vi "HEWH Setpoint Temperature Test Requriments.vi"(8 "error in":errorcluster, 11 "UEF Calculated Values Input":T1 {"Data Indexes"."15 sec after Draw Index" format="%#.2f"; "Data Indexes"."15 sec after Draw Timestamp" format="%#.2f"; "Data Indexes"."Test Start Timestamp" format="%.2f"; "Data Indexes"."Test End Timestamp" format="%.2f"; "Data Indexes"."T0 Timestamp" format="%.2f"; "Data Indexes"."Tsf Timestamp" format="%.2f"; "Data Indexes"."Tsu0 Timestamp" format="%.2f"; "Data Indexes"."Tmax1 Timestamp" format="%.2f"; "Data Indexes"."Draw Index Timestamp" format="%#.2f"; "Data Indexes"."Non-Draw Timestamp" format="%#.2f"; "Data Indexes"."Heating Timestamp" format="%#.2f"; "Data Indexes"."Start Energy (BTU-Gas)" format="%.6f"; "Data Indexes"."Start Watt Hours" format="%.6f"; "Static Data"."V - Volume of Wh (True)" format="%.5f"; "Static Data"."T-Ambinet Nominal (°F)" format="%.5f"; "Static Data"."T-Inlet Setpoint (°F)" format="%.5f"; "Static Data"."T-Wh Setpoint (°F)" format="%.5f"; "Sampled Data"."Qe (Wh)" format="%.5f"; "Sampled Data"."Tau stby2 (hr)" format="%.5f"; "Sampled Data"."Tastby2 (°F)" format="%.5f"; "Sampled Data"."Qf (BTU)" format="%.5f"; "Sampled Data"."Qe (BTU)" format="%.5f"; "Sampled Data"."Tmax1 (°F)" format="%.5f"; "Sampled Data"."T0 (°F)" format="%.5f"; "Sampled Data"."Qr (BTU)" format="%.5f"; "Sampled Data"."T 24(°F)" format="%.5f"; "Sampled Data"."T astby(°F)" format="%.5f"; "Sampled Data"."T tstby(°F)" format="%.5f"; "Sampled Data"."T su0(°F)" format="%.5f"; "Sampled Data"."T suf(°F)" format="%.5f"; "Sampled Data"."Tau stby_1 (hr)" format="%.5f"; "Sampled Data"."Qsuf (BTU)" format="%.5f"; "Sampled Data"."Qsu0 (BTU)" format="%.5f"; "Calculated Values"."Draw Bonus Volume (gal)" format="%.6f"; "Calculated Values"."Adjustment Factor" format="%.6f"; "Calculated Values"."T*avg_del(n-1)" format="%.6f"; "Calculated Values"."T*min(n-1)" format="%.6f"; "Calculated Values"."T*avg_del(n)" format="%.6f"; "Calculated Values"."Vn" format="%.6f"; "Calculated Values"."Qdm (BTU)" format="%.6f"; "Calculated Values"."QHWD (BTU)" format="%.6f"; "Calculated Values"."QHW (BTU)" format="%.6f"; "Calculated Values"."UEF" format="%.6f"; "Calculated Values"."QHW67 (BTU)" format="%.6f"; "Calculated Values"."Qda (BTU)" format="%.6f"; "Calculated Values"."Qd (BTU)" format="%.6f"; "Calculated Values"."Q (BTU)" format="%.6f"; "Calculated Values"."UA (BTU/(hr*F))" format="%.6f"; "Calculated Values"."Qhr (BTU/hr)" format="%.6f"; "Calculated Values"."Qstby (BTU)" format="%.6f"; "Calculated Values"."nu_r" format="%.6f"; "Calculated Values"."CpUEF (BTU/(lb*F))" format="%.6f"; "Calculated Values"."rho_nu (lb/gal)" format="%.6f"; "Calculated Values"."V1- Vol (Gal)" format="%.6f"; "Calculated Values"."M cluster mass removed (lb)" format="%.6f"; "Calculated Values"."Cp theoretical (BTU/(lbm °F))" format="%.6f"; "Calculated Values"."Tin1 - Mean Inlet 1st Cluster (°F)" format="%.6f"; "Calculated Values"."Tdel1-Mean Outlet 1st Cluster(°F)" format="%.6f"; "Calculated Values"."Cp 24 (BTU/(lb*F))" format="%.6f"; "Calculated Values"."Cp standby (BTU/(lb*F))" format="%.6f"; "Calculated Values"."Cp2 (BTU/(lb*F))" format="%.6f"; "Calculated Values"."Cp1 (BTU/(lb*F))" format="%.6f"; "Calculated Values"."rho 24 (lb/gal)" format="%.6f"; "Calculated Values"."rho standby (lb/gal)" format="%.6f"; "Calculated Values"."rho 2 (lb/gal)" format="%.6f"; "Calculated Values"."Density of cold water All (lbm/gal)" format="%#.3g"; "Calculated Values"."CpHW (BTU/(lbm °F))" format="%#.3g"; "Calculated Values"."Density of hot water All (lbm/gal)" format="%#.3g"; "Calculated Values"."Mass of water All (lbm)" format="%#.3f"}) -> (0 "error out":errorcluster, 3 "UEF Calculated Values Output":T1 {"Data Indexes"."15 sec after Draw Index" format="%#.2f"; "Data Indexes"."15 sec after Draw Timestamp" format="%#.2f"; "Data Indexes"."Test Start Timestamp" format="%.2f"; "Data Indexes"."Test End Timestamp" format="%.2f"; "Data Indexes"."T0 Timestamp" format="%.2f"; "Data Indexes"."Tsf Timestamp" format="%.2f"; "Data Indexes"."Tsu0 Timestamp" format="%.2f"; "Data Indexes"."Tmax1 Timestamp" format="%.2f"; "Data Indexes"."Draw Index Timestamp" format="%#.2f"; "Data Indexes"."Non-Draw Timestamp" format="%#.2f"; "Data Indexes"."Heating Timestamp" format="%#.2f"; "Data Indexes"."Start Energy (BTU-Gas)" format="%.6f"; "Data Indexes"."Start Watt Hours" format="%.6f"; "Static Data"."V - Volume of Wh (True)" format="%.5f"; "Static Data"."T-Ambinet Nominal (°F)" format="%.5f"; "Static Data"."T-Inlet Setpoint (°F)" format="%.5f"; "Static Data"."T-Wh Setpoint (°F)" format="%.5f"; "Sampled Data"."Qe (Wh)" format="%.5f"; "Sampled Data"."Tau stby2 (hr)" format="%.5f"; "Sampled Data"."Tastby2 (°F)" format="%.5f"; "Sampled Data"."Qf (BTU)" format="%.5f"; "Sampled Data"."Qe (BTU)" format="%.5f"; "Sampled Data"."Tmax1 (°F)" format="%.5f"; "Sampled Data"."T0 (°F)" format="%.5f"; "Sampled Data"."Qr (BTU)" format="%.5f"; "Sampled Data"."T 24(°F)" format="%.5f"; "Sampled Data"."T astby(°F)" format="%.5f"; "Sampled Data"."T tstby(°F)" format="%.5f"; "Sampled Data"."T su0(°F)" format="%.5f"; "Sampled Data"."T suf(°F)" format="%.5f"; "Sampled Data"."Tau stby_1 (hr)" format="%.5f"; "Sampled Data"."Qsuf (BTU)" format="%.5f"; "Sampled Data"."Qsu0 (BTU)" format="%.5f"; "Calculated Values"."Draw Bonus Volume (gal)" format="%.6f"; "Calculated Values"."Adjustment Factor" format="%.6f"; "Calculated Values"."T*avg_del(n-1)" format="%.6f"; "Calculated Values"."T*min(n-1)" format="%.6f"; "Calculated Values"."T*avg_del(n)" format="%.6f"; "Calculated Values"."Vn" format="%.6f"; "Calculated Values"."Qdm (BTU)" format="%.6f"; "Calculated Values"."QHWD (BTU)" format="%.6f"; "Calculated Values"."QHW (BTU)" format="%.6f"; "Calculated Values"."UEF" format="%.6f"; "Calculated Values"."QHW67 (BTU)" format="%.6f"; "Calculated Values"."Qda (BTU)" format="%.6f"; "Calculated Values"."Qd (BTU)" format="%.6f"; "Calculated Values"."Q (BTU)" format="%.6f"; "Calculated Values"."UA (BTU/(hr*F))" format="%.6f"; "Calculated Values"."Qhr (BTU/hr)" format="%.6f"; "Calculated Values"."Qstby (BTU)" format="%.6f"; "Calculated Values"."nu_r" format="%.6f"; "Calculated Values"."CpUEF (BTU/(lb*F))" format="%.6f"; "Calculated Values"."rho_nu (lb/gal)" format="%.6f"; "Calculated Values"."V1- Vol (Gal)" format="%.6f"; "Calculated Values"."M cluster mass removed (lb)" format="%.6f"; "Calculated Values"."Cp theoretical (BTU/(lbm °F))" format="%.6f"; "Calculated Values"."Tin1 - Mean Inlet 1st Cluster (°F)" format="%.6f"; "Calculated Values"."Tdel1-Mean Outlet 1st Cluster(°F)" format="%.6f"; "Calculated Values"."Cp 24 (BTU/(lb*F))" format="%.6f"; "Calculated Values"."Cp standby (BTU/(lb*F))" format="%.6f"; "Calculated Values"."Cp2 (BTU/(lb*F))" format="%.6f"; "Calculated Values"."Cp1 (BTU/(lb*F))" format="%.6f"; "Calculated Values"."rho 24 (lb/gal)" format="%.6f"; "Calculated Values"."rho standby (lb/gal)" format="%.6f"; "Calculated Values"."rho 2 (lb/gal)" format="%.6f"; "Calculated Values"."Density of cold water All (lbm/gal)" format="%#.3g"; "Calculated Values"."CpHW (BTU/(lbm °F))" format="%#.3g"; "Calculated Values"."Density of hot water All (lbm/gal)" format="%#.3g"; "Calculated Values"."Mass of water All (lbm)" format="%#.3f"})   [LabVIEW 2023]
uses:
  Type Definitions/UEF Constants.ctl
  Type Definitions/HEWH Draw Stats.ctl
  Type Definitions/HEWH FHR Draw Type.ctl
  Type Definitions/FHR Bins.ctl
  Type Definitions/HEWH Meter Type.ctl
  <vilib>/Utility/error.llb/whitespace.ctl
  <vilib>/Utility/error.llb/Trim Whitespace One-Sided.vi
panel:
  out "Array":string[][](array[string])
  out "ToutletMin":dbl[](array[numeric])
  out "ToutletMax":dbl[](array[numeric])
  # "FHR"
  # "FHR"
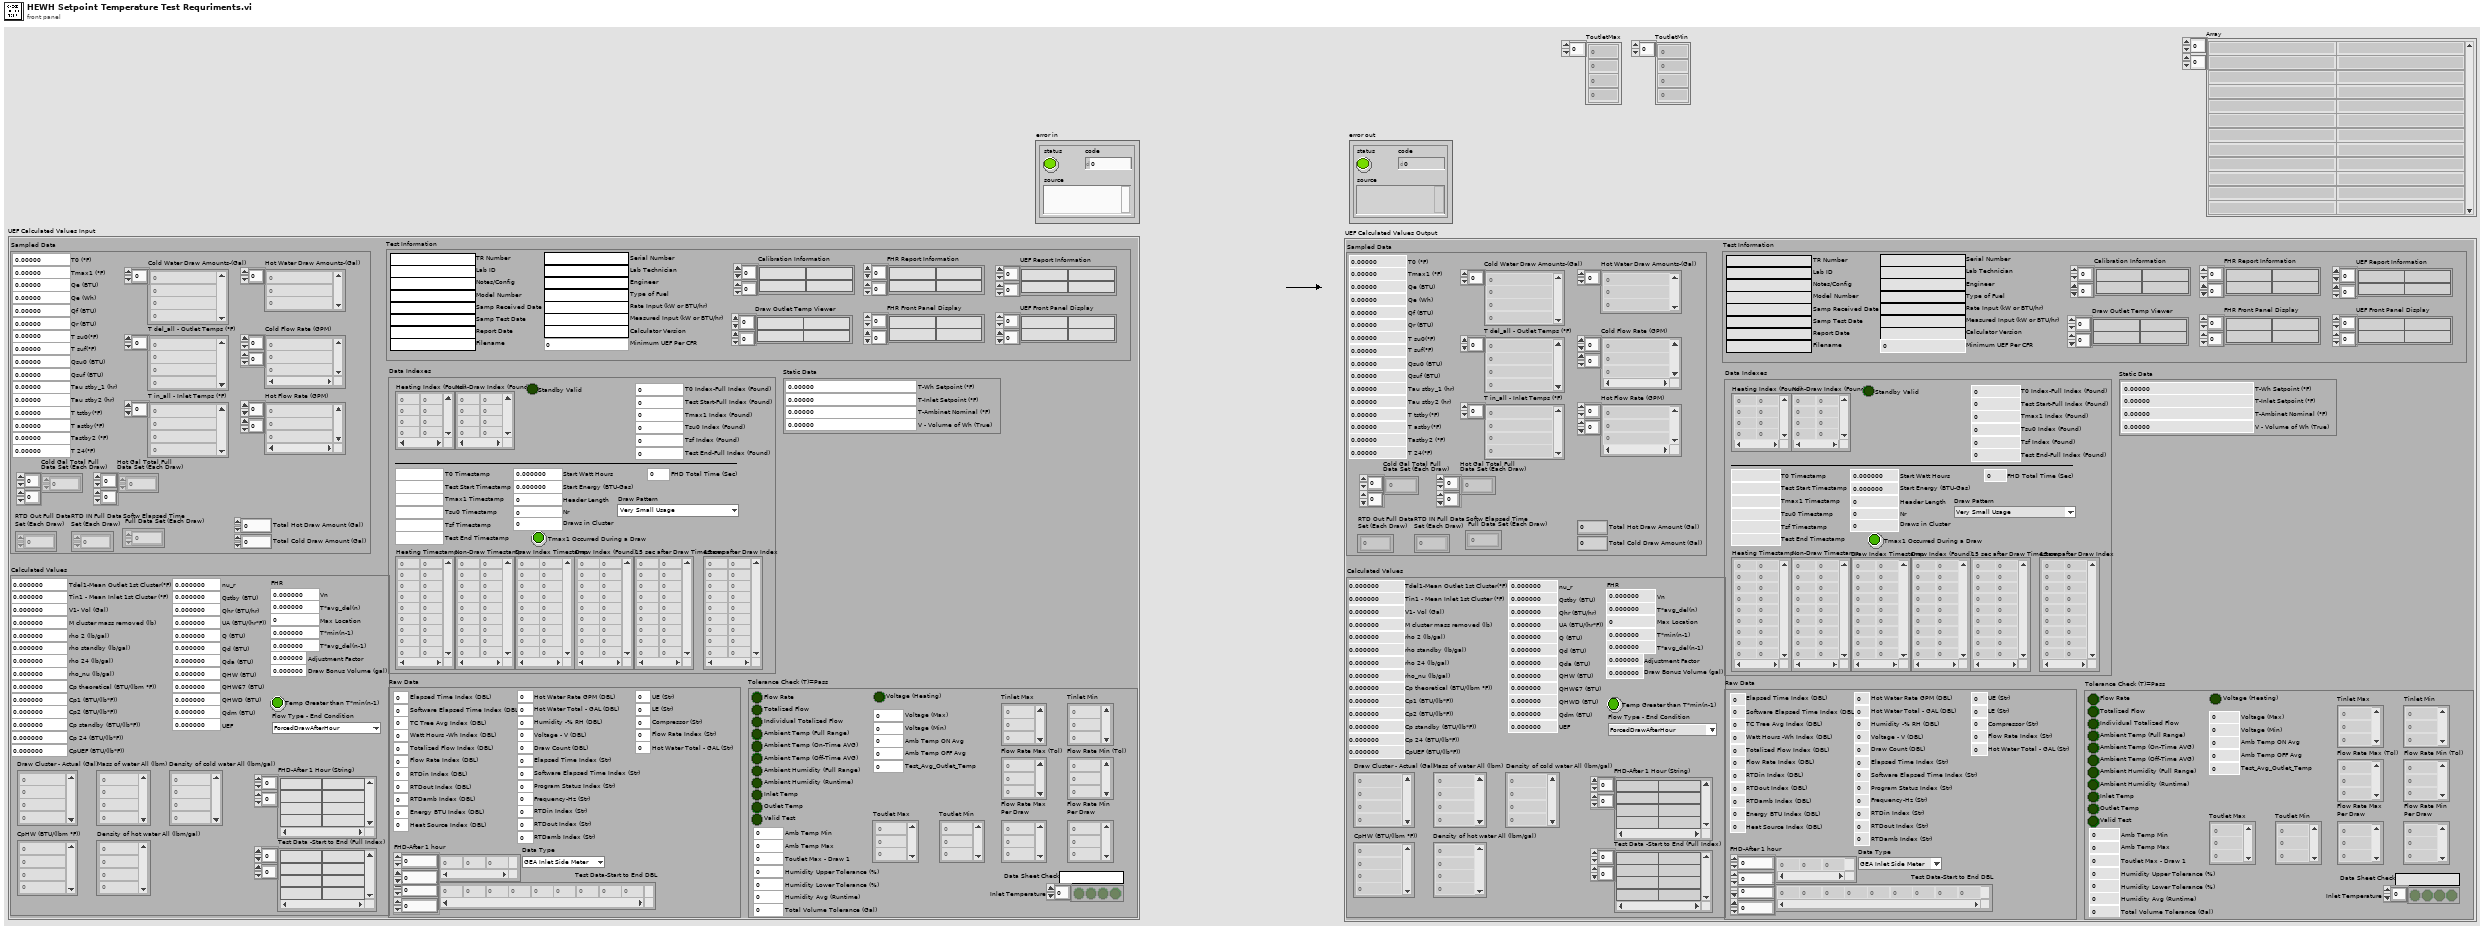
[diagram p1: front panel]
types:
  T1 = typedef "UEF Constants.ctl" = cluster{"Calculated Values":T2, "Sampled Data":cluster{"Cold Water Draw Amounts-(Gal)":dbl[], "T del_all - Outlet Temps (°F)":dbl[], "T in_all - Inlet Temps (°F)":dbl[], "Qsu0 (BTU)":dbl, "Qsuf (BTU)":dbl, "Tau stby_1 (hr)":dbl, "T suf(°F)":dbl, "T su0(°F)":dbl, "T tstby(°F)":dbl, "T astby(°F)":dbl, "T 24(°F)":dbl, "Qr (BTU)":dbl, "T0 (°F)":dbl, "Tmax1 (°F)":dbl, "Qe (BTU)":dbl, "Qf (BTU)":dbl, "Tastby2 (°F)":dbl, "RTD Out Full Data\nSet (Each Draw)":dbl[][], "RTD IN Full Data\nSet (Each Draw)":dbl[][], "Tau stby2 (hr)":dbl, "Hot Water Draw Amounts-(Gal)":dbl[], "Cold Flow Rate (GPM)":dbl[][], "Hot Flow Rate (GPM)":dbl[][], "Softw Elapsed Time\n Full Data Set (Each Draw)":dbl[][], "Cold Gal Total Full\nData Set (Each Draw)":dbl[][], "Total Hot Draw Amount (Gal) ":dbl, "Total Cold Draw Amount (Gal)":dbl, "Qe (Wh)":dbl, "Hot Gal Total Full\nData Set (Each Draw)":dbl[][]}, "Static Data":cluster{"T-Wh Setpoint (°F)":dbl, "T-Inlet Setpoint (°F)":dbl, "T-Ambinet Nominal (°F)":dbl, "V - Volume of Wh (True)":dbl}, "Data Indexes":cluster{"Test Start-Full Index (Found)":i32, "Header Length":i32, "Draw Index (Found)":i32[][], "Nr":i32, "Start Watt Hours":dbl, "Tsu0 Index (Found)":i32, "Tsf Index (Found)":i32, "Start Energy (BTU-Gas)":dbl, "Draws in Cluster":i32, "T0 Index-Full Index (Found)":i32, "Non-Draw Index (Found)":i32[][], "Tmax1 Index (Found)":i32, "Test End-Full Index (Found)":i32, "Heating Index (Found)":i32[][], "Heating Timestamp":dbl[][], "Non-Draw Timestamp":dbl[][], "Draw Index Timestamp":dbl[][], "Tmax1 Timestamp":dbl, "Tsu0 Timestamp":dbl, "Tsf Timestamp":dbl, "T0 Timestamp":dbl, "Test End Timestamp":dbl, "Test Start Timestamp":dbl, "15 sec after Draw Timestamp":dbl[][], "15 sec after Draw Index":dbl[][], "Tmax1 Occurred During a Draw":bool, "FHD Total Time (Sec)":dbl, "Draw Pattern":T4, "Standby Valid":bool}, "Raw Data":cluster{"Elapsed Time Index (DBL)":i32, "Software Elapsed Time Index (DBL)":i32, "TC Tree Avg Index (DBL)":i32, "Watt Hours -Wh Index (DBL)":i32, "Energy BTU Index (DBL)":i32, "Totalized Flow Index (DBL)":i32, "Flow Rate Index (DBL)":i32, "Program Status Index (Str)":i32, "RTDin Index (DBL)":i32, "RTDout Index (DBL)":i32, "RTDamb Index (DBL)":i32, "Test Data-Start to End DBL":dbl[][], "Data Type":T5, "Heat Source Index (DBL)":i32, "Hot Water Rate GPM (DBL)":i32, "Hot Water Total - GAL (DBL)":i32, "FHD-After 1 hour":dbl[][], "Humidity -% RH (DBL)":i32, "Voltage - V (DBL)":i32, "Draw Count (DBL)":i32, "Elapsed Time Index (Str)":i32, "Software Elapsed Time Index (Str)":i32, "Frequency-Hz (Str)":i32, "RTDin Index (Str)":i32, "RTDout Index (Str)":i32, "RTDamb Index (Str)":i32, "UE (Str)":i32, "LE (Str)":i32, "Compressor (Str)":i32, "Flow Rate Index (Str)":i32, "Hot Water Total - GAL (Str)":i32}, "Tolerance Check (T)=Pass":cluster{"Flow Rate":bool, "Totalized Flow":bool, "Ambient Temp (Full Range)":bool, "Ambient Humidity (Full Range)":bool, "Inlet Temp":bool, "Outlet Temp":bool, "Valid Test":bool, "Individual Totalized Flow":bool, "Data Sheet Check":string, "Inlet Temperature":bool[], "Tinlet Max":dbl[], "Tinlet Min":dbl[], "Flow Rate Max (Tol)":dbl[], "Flow Rate Min (Tol)":dbl[], "Amb Temp Max":dbl, "Amb Temp Min":dbl, "Toutlet Max - Draw 1":dbl, "Humidity Upper Tolerance (%)":dbl, "Total Volume Tolerance (Gal)":dbl, "Humidity Lower Tolerance (%)":dbl, "Flow Rate Max\nPer Draw":dbl[], "Flow Rate Min\nPer Draw":dbl[], "Ambient Humidity (Runtime)":bool, "Humidity Avg (Runtime)":dbl, "Ambient Temp (On-Time AVG)":bool, "Ambient Temp (Off-Time AVG)":bool, "Amb Temp OFF Avg":dbl, "Amb Temp ON Avg":dbl, "Voltage (Heating)":bool, "Voltage (Min)":dbl, "Voltage (Max)":dbl, "Toutlet Max":dbl[], "Toutlet Min":dbl[], "Test_Avg_Outlet_Temp":dbl}, "Test Information":cluster{"TR Number":string, "Lab ID":string, "Notes/Config":string, "Model Number":string, "Serial Number":string, "Lab Technician":string, "Engineer":string, "Type of Fuel":string, "Samp Received Date":string, "Samp Test Date":string, "Report Date":string, "Rate Input (kW or BTU/hr)":string, "Measured Input (kW or BTU/hr)":string, "Filename":string, "Calibration Information":string[][], "Calculator Version":string, "Minimum UEF Per CFR":dbl, "UEF Report Information":string[][], "FHR Report Information":string[][], "FHR Front Panel Display":string[][], "UEF Front Panel Display":string[][], "Draw Outlet Temp Viewer":string[][]}}
  T2 = typedef "HEWH Draw Stats.ctl" = cluster{"Draw Cluster - Actual (Gal)":dbl[], "Mass of water All (lbm)":dbl[], "Density of hot water All (lbm/gal)":dbl[], "CpHW (BTU/(lbm °F))":dbl[], "rho 2 (lb/gal)":dbl, "rho standby (lb/gal)":dbl, "rho 24 (lb/gal)":dbl, "Cp1 (BTU/(lb*F))":dbl, "Cp2 (BTU/(lb*F))":dbl, "Cp standby (BTU/(lb*F))":dbl, "Cp 24 (BTU/(lb*F))":dbl, "nu_r":dbl, "Qstby (BTU)":dbl, "Qhr (BTU/hr)":dbl, "UA (BTU/(hr*F))":dbl, "Q (BTU)":dbl, "Qd (BTU)":dbl, "Qda (BTU)":dbl, "QHW67 (BTU)":dbl, "UEF":dbl, "Tdel1-Mean Outlet 1st Cluster(°F)":dbl, "Tin1 - Mean Inlet 1st Cluster (°F)":dbl, "Cp theoretical (BTU/(lbm °F))":dbl, "M cluster mass removed (lb)":dbl, "V1- Vol (Gal)":dbl, "Test Data -Start to End (Full Index)":string[][], "rho_nu (lb/gal)":dbl, "Density of cold water All (lbm/gal)":dbl[], "CpUEF (BTU/(lb*F))":dbl, "QHW (BTU)":dbl, "QHWD (BTU)":dbl, "Qdm (BTU)":dbl, "FHD-After 1 Hour (String)":string[][], "Vn":dbl, "T*avg_del(n)":dbl, "Max Location":i32, "T*min(n-1)":dbl, "T*avg_del(n-1)":dbl, "Temp Greater than T*min(n-1)":bool, "Adjustment Factor":dbl, "Draw Bonus Volume (gal)":dbl, "Flow Type - End Condition":T3}
  T3 = typedef "HEWH FHR Draw Type.ctl" = enum16{"ForcedDrawAfterHour", "HeatingCutoffBeforeHour"}
  T4 = typedef "FHR Bins.ctl" = enum16{"Very Small Usage", "Low Usage", "Medium Usage", "High Usage", "Undefined"}
  T5 = typedef "HEWH Meter Type.ctl" = enum16{"GEA Inlet Side Meter", "GEA Outlet Side Meter", "CSA Inlet Side Meter"}
  T6 = typedef "whitespace.ctl" = u16
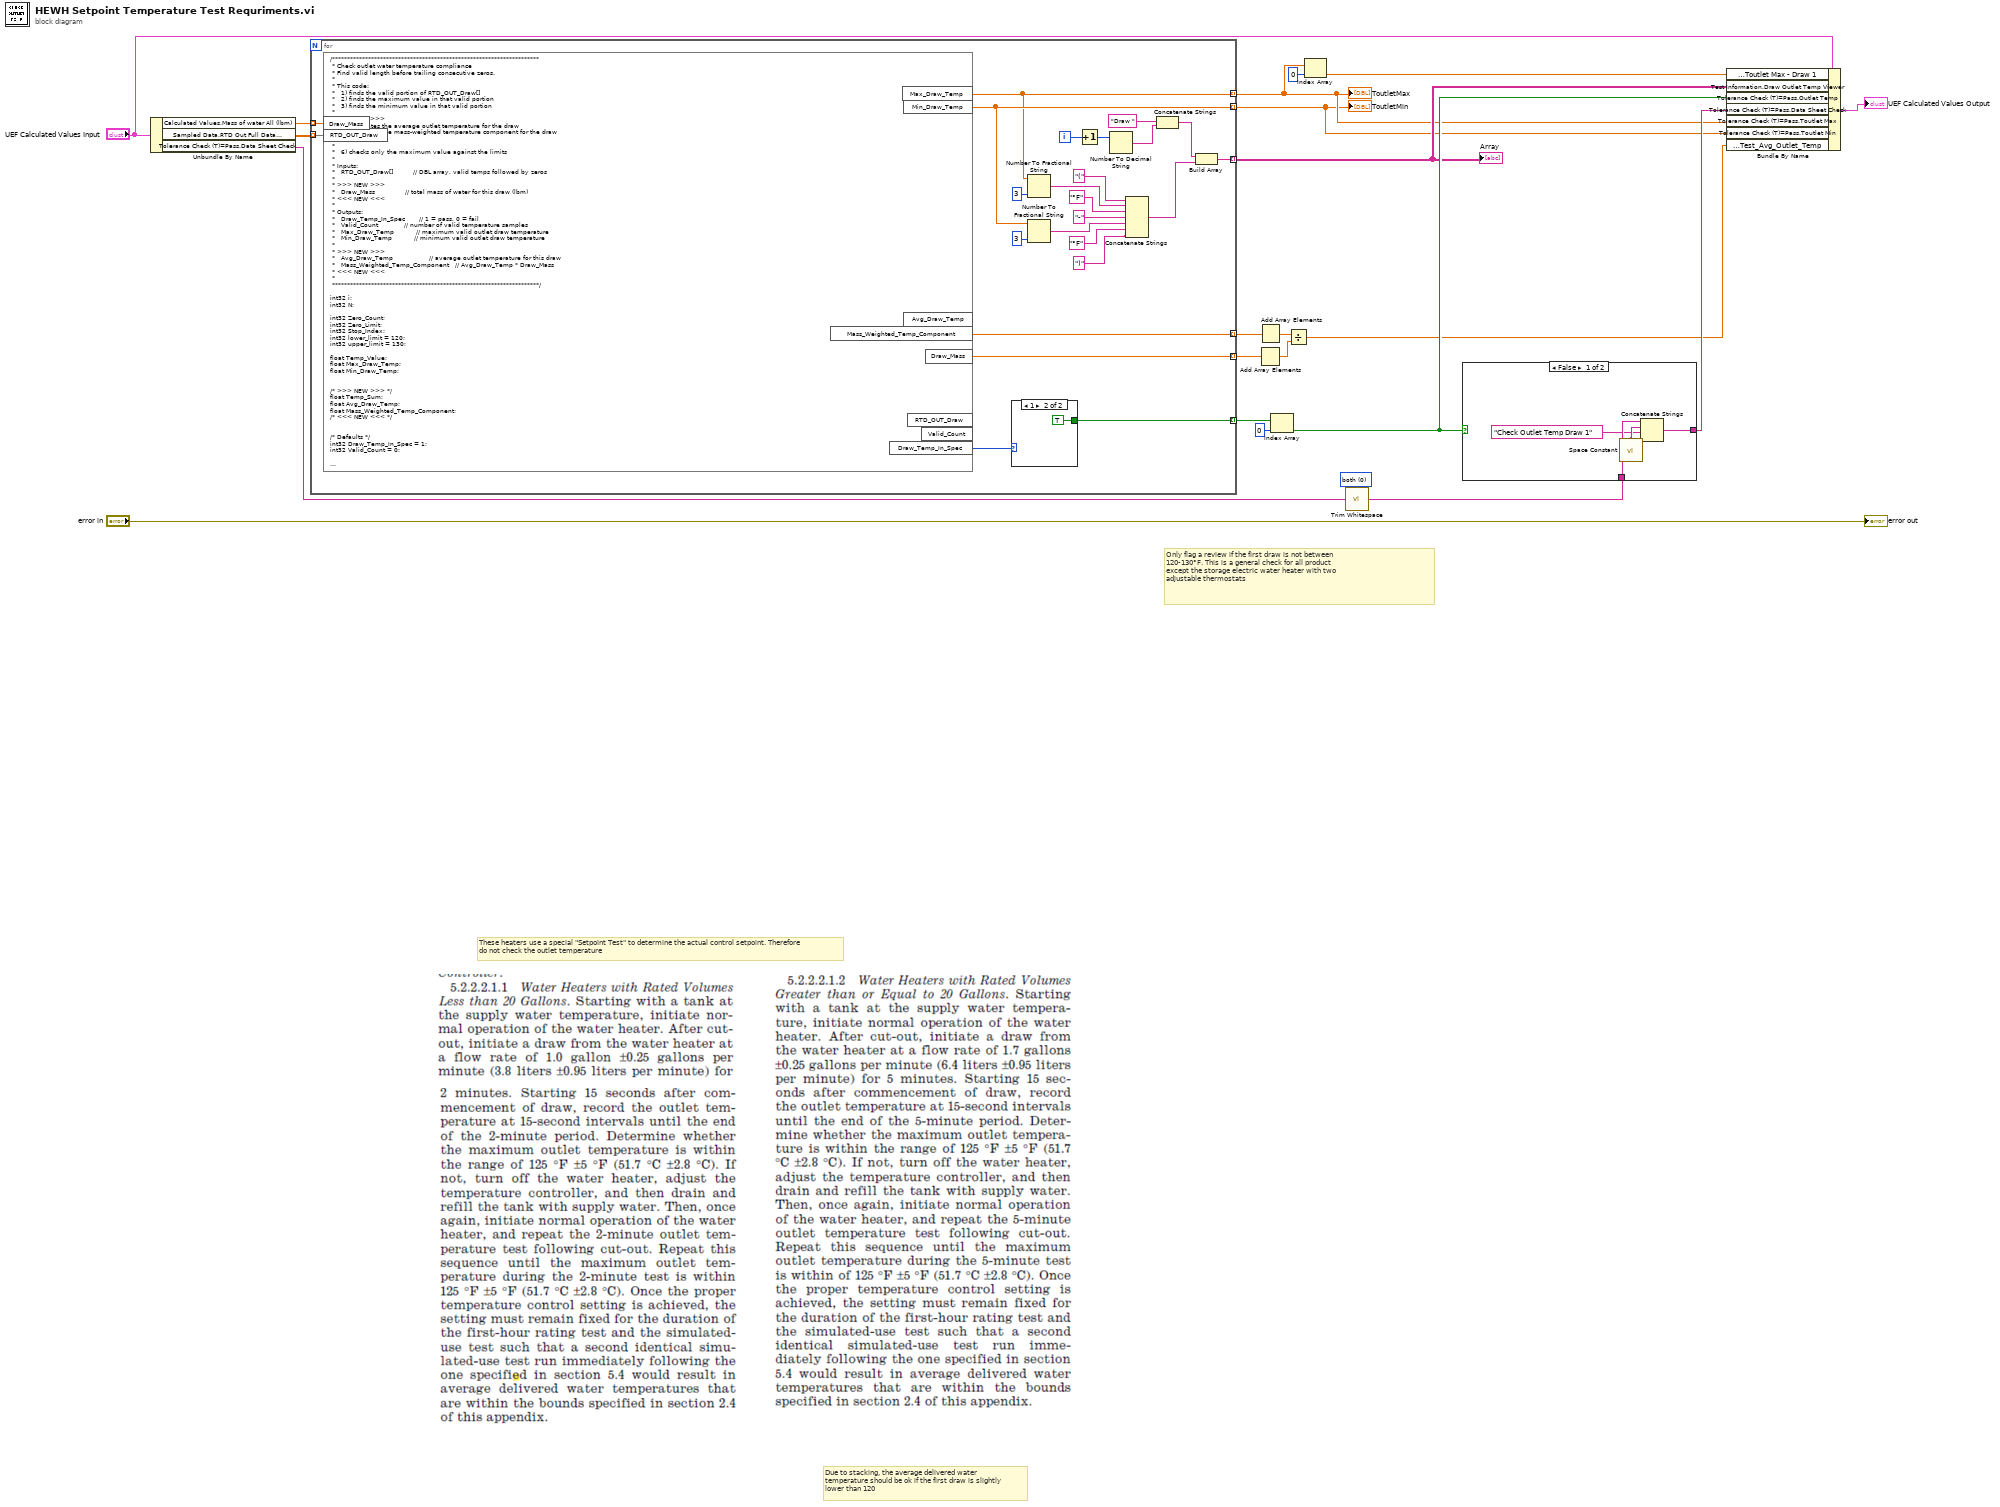
[diagram p0: block diagram]
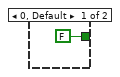
[diagram p3: hidden frame]
diagram:
  w11 = T6 0 items=["both", "start of string", "end of string"] ("location (both)")
  # "Only flag a review if the first draw is not between\n120-130°F. This is a general check for all product\nexcept the storage electric water heater with two \nadjustable thermostats"
  # "These heaters use a special \"Setpoint Test\" to determine the actual control setpoint. Therefore\ndo not check the outlet temperature"
  # "Due to stacking, the average delivered water\ntemperature should be ok if the first draw is slightly \nlower than 120"
  n1 = Unbundle By Name("UEF Calculated Values Input") -> ("Calculated Values.Mass of water All (lbm)"=w6:dbl[], "Sampled Data.RTD Out Full Data\nSet (Each Draw)"=w18:dbl[][], "Tolerance Check (T)=Pass.Data Sheet Check"=w13:string)
  n2 = for {
    tunnel: w18 -> [w30] mode=indexing
    tunnel: [w35] -> w9 mode=indexing
    tunnel: [w28] -> w20 mode=indexing
    tunnel: [w26] -> w8 mode=indexing
    tunnel: [w27] -> w7 mode=indexing
    tunnel: w6 -> [w25] mode=indexing
    tunnel: [w24] -> w5 mode=indexing
    tunnel: [w23] -> w3 mode=indexing
    i -> [w34]
    n3 = formula code="/*********************************************************************\n * Check outlet water temperature compliance\n * Find valid length before trailing consecutive zeros.\n *\n * This code:\n *   1) finds the valid portion of RTD_OUT_Draw[]\n *   2) finds the maximum value in that valid portion\n *   3) finds the minimum value in that valid portion\n *\n * >>> NEW >>>\n *   4) calculates the average outlet temperature for the draw\n *   5) calculates the mass-weighted temperature component for the draw\n * <<< NEW <<<\n *\n *   6) checks only the maximum value against the limits\n *\n * Inputs:\n *   RTD_OUT_Draw[]          // DBL array, valid temps followed by zeros\n *\n * >>> NEW >>>\n *   Draw_Mass               // total mass of water for this draw (lbm)\n * <<< NEW <<<\n *\n * Outputs:\n *   Draw_Temp_In_Spec       // 1 = pass, 0 = fail\n *   Valid_Count             // number of valid temperature samples\n *   Max_Draw_Temp           // maximum valid outlet draw temperature\n *   Min_Draw_Temp           // minimum valid outlet draw temperature\n *\n * >>> NEW >>>\n *   Avg_Draw_Temp                  // average outlet temperature for this draw\n *   Mass_Weighted_Temp_Component   // Avg_Draw_Temp * Draw_Mass\n * <<< NEW <<<\n *\n *********************************************************************/\n\nint32 i;\nint32 N;\n\nint32 Zero_Count;\nint32 Zero_Limit;\nint32 Stop_Index;\nint32 lower_limit = 120;\nint32 upper_limit = 130;\n\nfloat Temp_Value;\nfloat Max_Draw_Temp;\nfloat Min_Draw_Temp;\n\n\n/* >>> NEW >>> */\nfloat Temp_Sum;\nfloat Avg_Draw_Temp;\nfloat Mass_Weighted_Temp_Component;\n/* <<< NEW <<< */\n\n\n/* Defaults */\nint32 Draw_Temp_In_Spec = 1;\nint32 Valid_Count = 0;\n\n\n/* >>> NEW >>> */\nTemp_Sum = 0.0;\nAvg_Draw_Temp = 0.0;\nMass_Weighted_Temp_Component = 0.0;\n/* <<< NEW <<< */\n\n\nZero_Count = 0;\nZero_Limit = 3;        /* Stop after 3 consecutive zeros */\nStop_Index = -1;\n\nN = sizeOfDim(RTD_OUT_Draw, 0);\n\n\n/*\n * Find the start of the trailing zero section.\n */\nfor (i = 0; i < N; i++)\n{\n    Temp_Value = RTD_OUT_Draw[i];\n\n    if (Temp_Value == 0.0)\n    {\n        Zero_Count += 1;\n\n        if (Zero_Count >= Zero_Limit)\n        {\n            /*\n             * i is the index of the third zero.\n             * Last valid temp is before the zero run.\n             */\n            Stop_Index = i - Zero_Limit;\n            break;\n        }\n    }\n    else\n    {\n        Zero_Count = 0;\n    }\n}\n\n\n/*\n * If no trailing zero section was found, use the full array.\n */\nif (Stop_Index < 0)\n{\n    Stop_Index = N - 1;\n}\n\n\n/*\n * Number of valid samples to keep.\n */\nValid_Count = Stop_Index + 1;\n\n\n/*\n * Find the maximum and minimum valid temperatures.\n * Only the maximum temperature is checked against the limits.\n */\nif (Valid_Count > 0)\n{\n    Max_Draw_Temp = RTD_OUT_Draw[0];\n    Min_Draw_Temp = RTD_OUT_Draw[0];\n\n\n    /* >>> NEW >>> */\n    /*\n     * Start the temperature sum with the first valid sample.\n     */\n    Temp_Sum = RTD_OUT_Draw[0];\n    /* <<< NEW <<< */\n\n\n    for (i = 1; i < Valid_Count; i++)\n    {\n        Temp_Value = RTD_OUT_Draw[i];\n\n\n        /* >>> NEW >>> */\n        /*\n         * Add each valid temperature sample to the running sum.\n         */\n        Temp_Sum += Temp_Value;\n        /* <<< NEW <<< */\n\n\n        if (Temp_Value > Max_Draw_Temp)\n        {\n            Max_Draw_Temp = Temp_Value;\n        }\n\n        if (Temp_Value < Min_Draw_Temp)\n        {\n            Min_Draw_Temp = Temp_Value;\n        }\n    }\n\n\n    /* >>> NEW >>> */\n    /*\n     * Calculate average outlet temperature for this draw.\n     */\n    Avg_Draw_Temp = Temp_Sum / Valid_Count;\n\n\n    /*\n     * Calculate this draw's contribution to the whole-test\n     * mass-weighted average outlet temperature.\n     *\n     * Final calculation outside the For Loop:\n     *\n     *                       Sum(Mass_Weighted_Temp_Component)\n     * Test_Avg_Temp = -----------------------------------------\n     *                              Sum(Draw_Mass)\n     */\n    if (Draw_Mass > 0.0)\n    {\n        Mass_Weighted_Temp_Component =\n            Avg_Draw_Temp * Draw_Mass;\n    }\n    else\n    {\n        Mass_Weighted_Temp_Component = 0.0;\n    }\n    /* <<< NEW <<< */\n\n\n    if (Max_Draw_Temp < lower_limit || Max_Draw_Temp > upper_limit)\n    {\n        Draw_Temp_In_Spec = 0;\n    }\n}\nelse\n{\n    Max_Draw_Temp = 0.0;\n    Min_Draw_Temp = 0.0;\n\n\n    /* >>> NEW >>> */\n    Avg_Draw_Temp = 0.0;\n    Mass_Weighted_Temp_Component = 0.0;\n    /* <<< NEW <<< */\n\n\n    Draw_Temp_In_Spec = 0;\n}"("RTD_OUT_Draw"=w30, "Draw_Mass"=w25) -> ("Draw_Temp_In_Spec"=w29:i32, "Max_Draw_Temp"=w26:dbl, "Min_Draw_Temp"=w27:dbl, "Mass_Weighted_Temp_Component"=w24:dbl, "Draw_Mass"=w23:dbl)  [unwired: 3 out]
    n4 = case shown="1" w29 {
      tunnel: [FALSE TRUE] -> w28
      frame 0, Default {
      }
      frame 1 {
      }
    }
    n5 = Number To Fractional String(number=w26, precision (6)=i16 3) -> (F-format string=w46:string)  [unwired: 2 in]
    n6 = Number To Fractional String(number=w27, precision (6)=i16 3) -> (F-format string=w44:string)  [unwired: 2 in]
    n7 = Increment(x=w34) -> (x+1=w33:i32)
    n8 = Number To Decimal String(number=w33) -> (decimal integer string=w38:string)  [unwired: 1 in]
    n9 = Concatenate Strings("(" ("string"), w46, "°F" ("string"), "-" ("string"), w44, "°F" ("string"), ")" ("string")) -> (w36:string)
    n10 = Concatenate Strings("Draw ", w38) -> (w37:string)
    n11 = Build Array(w37, w36) -> (w35:string[])
  }
  "ToutletMax" <- w8
  "ToutletMin" <- w7
  "Array" <- w9
  n12 = Add Array Elements(numeric array=w3) -> (sum=w2:dbl)
  n13 = Add Array Elements(numeric array=w5) -> (sum=w4:dbl)
  n14 = Index Array(array=w20, index=0) -> (element=w10:bool)
  n15 = Divide(x=w4, y=w2) -> (x/y=w1:dbl)
  n16 = Index Array(array=w8, index=0) -> (element=w17:dbl)
  n17 = call <vilib>:"Trim Whitespace.vi"("string"=w13, "location (both)"=w11) -> ("trimmed string"=w12:string)
  n18 = case shown="False" w10 {
    tunnel: w12 -> [w51 w53]
    tunnel: [w49 w53] -> w14
    frame False {
      n19 = call <vilib>:"Space Constant.vi"() -> ("String"=w52:string)
      n20 = Concatenate Strings(w51, w52, "Check Outlet Temp Draw 1", w52) -> (w49:string)
    }
    frame True {
    }
  }
  n21 = Bundle By Name(cluster="UEF Calculated Values Input", "Tolerance Check (T)=Pass.Toutlet Max - Draw 1"=w17, "Test Information.Draw Outlet Temp Viewer"=w9, "Tolerance Check (T)=Pass.Outlet Temp"=w10, "Tolerance Check (T)=Pass.Data Sheet Check"=w14, "Tolerance Check (T)=Pass.Toutlet Max"=w8, "Tolerance Check (T)=Pass.Toutlet Min"=w7, "Tolerance Check (T)=Pass.Test_Avg_Outlet_Temp"=w1) -> (→"UEF Calculated Values Output":T1)
  "error out" <- "error in"
